vi "Basic upload example .vi"() -> ()   [LabVIEW 2013, in "Rinocloud Library.lvlib"]
uses:
  Rinocloud Library.lvlib
  <vilib>/Utility/file.llb/Write To Spreadsheet File (DBL).vi
  <vilib>/Analysis/NI_AALBase.lvlib
panel:
  in  "Refresh":bool
  out "Waveform Chart":dbl[](graph)
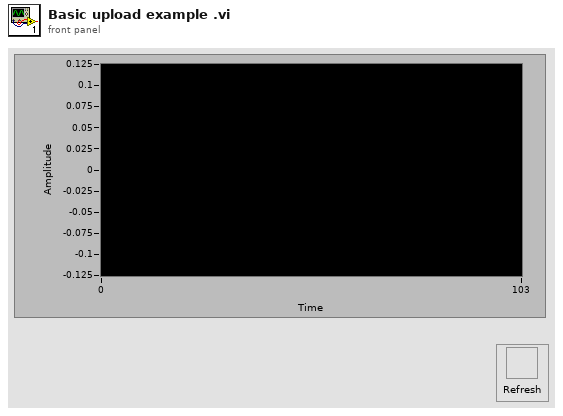
[diagram p1: front panel]
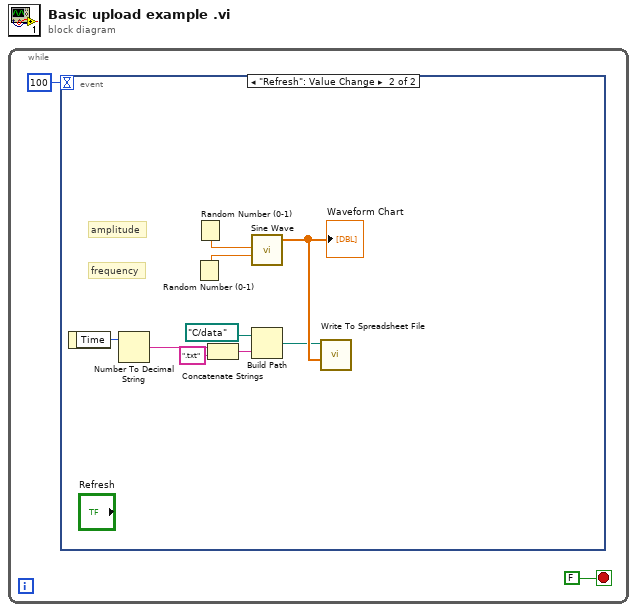
[diagram p0: block diagram]
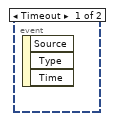
[diagram p2: hidden frame]
diagram:
  n1 = while {
    stop <- FALSE stop-if-true
    n2 = event shown="[1] \"Refresh\": Value Change" {
      selector: _ -> [_ _]
      dyn-events: _ -> [_ _]
      timeout: 100 -> [_ _]
      event Timeout {
        n3 = event-data() -> ()  [unwired: 1 in, 3 out]
      }
      event "Refresh": Value Change {
        # "frequency"
        # "amplitude"
        n4 = event-data() -> ("Time"=w7:u32)  [unwired: 1 in]
        n5 = Number To Decimal String(number=w7) -> (decimal integer string=w6:string)  [unwired: 1 in]
        n6 = Random Number (0-1)() -> (number: 0 to 1=w11:dbl)
        n7 = Random Number (0-1)() -> (number: 0 to 1=w3:dbl)
        n8 = Concatenate Strings(w6, ".txt" ("string")) -> (w4:string)
        n9 = call <vilib>:"Sine Wave.vi"("amplitude"=w3, "frequency"=w11) -> ("sine wave"=w10:dbl[])  [unwired: 3 in, 2 out]
        "Waveform Chart" <- w10
        n10 = Build Path(base path=path "C:/data" ("file path (dialog if empty)"), name or relative path=w4) -> (appended path=w8:path)
        n11 = call-poly <vilib>:"Write To Spreadsheet File.vi"("1D data"=w10, "file path (dialog if empty)"=w8) -> ()  [unwired: 6 in, 1 out]
      }
    }
  }
